vi "Acquisition-Counts error reporter.vi"(9 "Timed out waiting for expected number of acquisition points":bool, 11 "Counts cluster":T1) -> ()   [LabVIEW 2013]
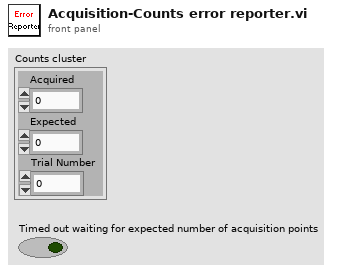
[diagram p1: front panel]
types:
  T1 = cluster{"Acquired":u32, "Expected":i32, "Trial Number":i32}
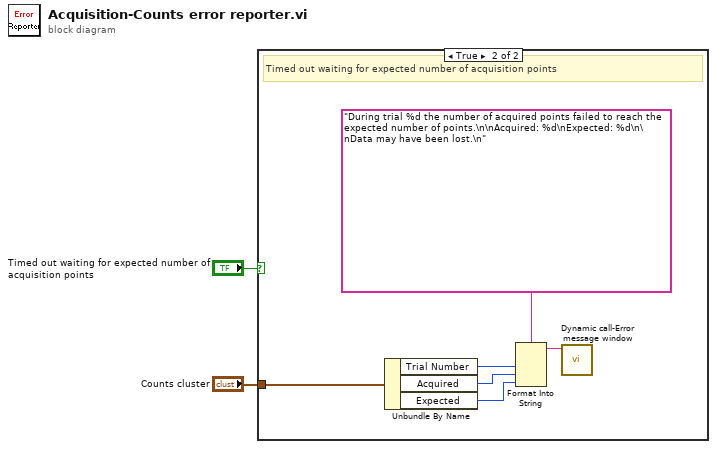
[diagram p0: block diagram]
diagram:
  n1 = case shown="True" "Timed out waiting for expected number of acquisition points" {
    tunnel: "Counts cluster" -> [_ w8]
    frame False {
      # "No timeout"
    }
    frame True {
      # "Timed out waiting for expected number of acquisition points"
      n2 = Unbundle By Name(w8) -> ("Trial Number"=w6:i32, "Acquired"=w5:u32, "Expected"=w4:i32)
      n3 = Format Into String(format string="During trial %d the number of acquired points failed to reach the expected number of points.\n\nAcquired: %d\nExpected: %d\n\nData may have been lost.\n", w6, w5, w4) -> (resulting string=w3:string)  [unwired: 2 in, 1 out]
      n4 = call "Dynamic call-Error message window.vi"("Error Message"=w3) -> ()  [unwired: 10 in, 1 out]
    }
  }
